vi "Msg.Q.Dequeue.vi"(6 "Dequeue Mode":T1, 8 "Error (in)":errorcluster, 11 "Msg.Q.Ref (in)":T2) -> (0 "Error (out)":errorcluster, 1 "Data":variant, 2 "Message":string, 3 "Msg.Q.Ref (out)":T2)   [LabVIEW 2023, in "MessagingModule.lvlib"]
doc: "This VI is used to dequeue message and data."
uses:
  Msg.Q.Ref.ctl
  Msg.Data.ctl
  Msg.Q.DequeueMode.ctl
  MessagingModule.lvlib
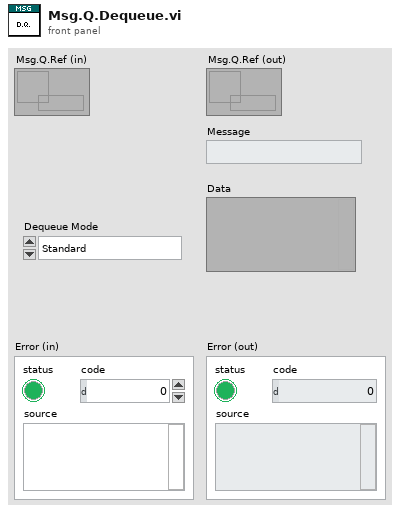
[diagram p1: front panel]
types:
  T1 = typedef "MessagingModule.lvlib/Msg.Q.DequeueMode.ctl" = enum16{"Standard", "Preview"}
  T2 = typedef "MessagingModule.lvlib/Msg.Q.Ref.ctl" = refnum<queue>
  T3 = typedef "MessagingModule.lvlib/Msg.Data.ctl" = cluster{"Message":string, "Data":variant}
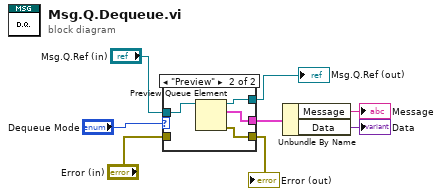
[diagram p0: block diagram]
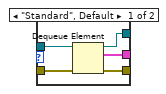
[diagram p2: hidden frame]
diagram:
  n1 = case shown="\"Preview\"" "Dequeue Mode" {
    tunnel: "Msg.Q.Ref (in)" -> [w13 w16]
    tunnel: "Error (in)" -> [w12 _]
    tunnel: [w11 w17] -> w6
    tunnel: [w10 w15] -> w5
    tunnel: [w9 w14] -> w4
    frame "Standard", Default {
      n2 = Dequeue Element(queue=w13, error in (no error)=w12) -> (queue out=w10:T2, element=w9:T3, error out=w11:errorcluster)  [unwired: 1 in, 1 out]
    }
    frame "Preview" {
      n3 = Preview Queue Element(queue=w16) -> (queue out=w15:T2, element=w14:T3, error out=w17:errorcluster)  [unwired: 2 in, 1 out]
    }
  }
  "Msg.Q.Ref (out)" <- w5
  "Error (out)" <- w6
  n4 = Unbundle By Name(w4) -> ("Message"=→"Message":string, "Data"=→"Data":variant)
